vi "sub2 swap.vi"(5 "Y":i32, 6 "X":i32, 7 "Original":dbl[](array[numeric])) -> (3 "After Swapped":dbl[](array[numeric]))   [LabVIEW 2014]
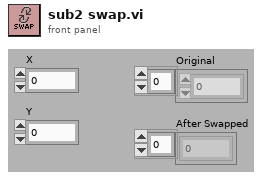
[diagram p1: front panel]
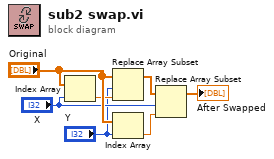
[diagram p0: block diagram]
diagram:
  n1 = Index Array(array="Original", index="X") -> (element=w6:dbl)
  n2 = Replace Array Subset(array="Original", new element=w6, index="Y") -> (w1:dbl[])
  n3 = Index Array(array="Original", index="Y") -> (element=w5:dbl)
  n4 = Replace Array Subset(array=w1, new element=w5, index="X") -> (→"After Swapped":dbl[])
